vi "TARGET.vi"() -> ()   [LabVIEW 2018]
uses:
  <vilib>/Platform/TimedLoop/XDataNode/timing_clust.ctl
  <vilib>/Platform/TimedLoop/XDataNode/nitl_modes.ctl
  <vilib>/Platform/TimedLoop/XDataNode/wakeup.ctl
  <vilib>/rvi/eio/common/nirviEmuTemplateMethod_errors.vi
  <vilib>/rvi/Emulation/niFpgaGetClockAttributes.vi
  <vilib>/rvi/Emulation/niFpgaSctlEmulationGetInTimedLoop.vi
  <vilib>/rvi/Emulation/niFpgaEmulationReportErrorSimple.vi
  <vilib>/rvi/Emulation/niFpgaCriticalErrorInLSC.vi
  <vilib>/rvi/interface/RandomDataEmulation/niFpgaRandomDataHandleErrors.vi
  <vilib>/rvi/Emulation/niFpgaProcessEmulError.vi
  <vilib>/eio/EIONode/EIONode.xnode
  <vilib>/Platform/TimedLoop/XDataNode/XDataNode.xnode
  <vilib>/rvi/DataTransferAndStorage/Container/XNode/niFpgaContainer.xnode
  <vilib>/rvi/interface/RandomDataEmulation/nirviRandomDataFpgaReadWriteTemplate.vi
  <vilib>/Platform/TimedLoop/XDataNode/XDNodeRunTimeDep.lvlib
panel:
  in  "IO Module\\Local_Supply_Select":u8
  in  "IO Module\\DDCA_Supply_Select":bool=TRUE
  in  "8191?":u16=8191
  in  "Задержка, мкс":u16 caption="Count(mSec)"
  in  "50?":u16=50
  in  "Запись в FIFO":bool
  in  "HIGH":u8=18
  in  "LOW":u8=8
  in  "CLK_1":u16=59
  in  "ROG_1":u16=20
  in  "ROG_2":u16=40
  in  "SHUT1":u16=95
  in  "SHUT_2":u16=125
  in  "CLK_2":u8=9
  in  "CLK_3":u8=20
  in  "20":u8=20
  in  "42000?":u16=42000
  in  "П_41789?":u16=41789
  in  "ADC_2":u8=13
  in  "ADC_1":u8=2
  in  "CDS2_2":u8=15
  in  "CDS2_1":u8=10
  in  "CDS1_2":u8=9
  in  "CDS1_1":u8=2
  out "Данные":u8
  in  "Направление бит":bool
  in  "Линейки":bool
  in  "Остановка основного цикла":bool
  in  "Command array":bool[](array[boolean])=[FALSE, FALSE, FALSE, FALSE, FALSE, FALSE, FALSE, FALSE, FALSE, FALSE, FALSE, FALSE, FALSE, FALSE, FALSE, FALSE, FALSE]
  in  "Read(T)/Write(F)":bool
  in  "Enum":T1(ring)=enum."GREEN PGA"
  in  "Write Data":bool[](array[boolean])=[FALSE, FALSE, FALSE, FALSE, FALSE, FALSE, FALSE, FALSE, FALSE]
  out "READ":bool[](array[boolean])
  in  "Конфигурация":bool
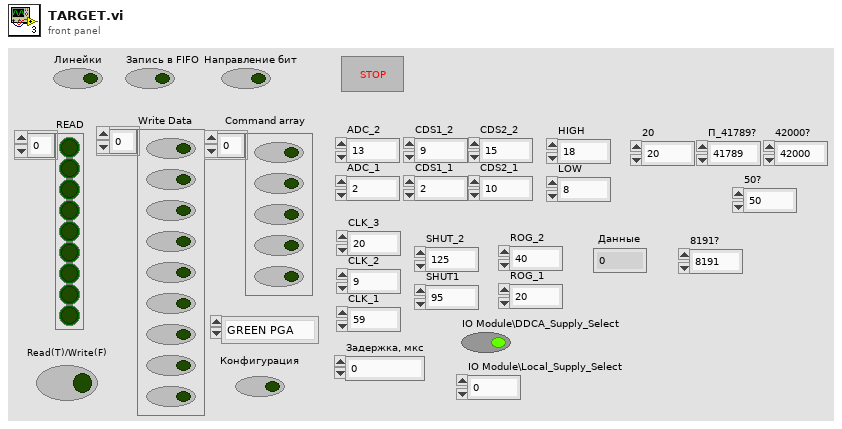
[diagram p1: front panel]
types:
  T1 = enum16{"Configuration", "MUX", "RED PGA", "GREEN PGA", "BLUE PGA", "RED OFF", "GREEN OFF", "BLUE OFF"}
  T2 = typedef "XDNodeRunTimeDep.lvlib/timing_clust.ctl" = cluster{"Expected End [f-1]":u64, "Actual End [f-1]":u64, "Finished Late? [f-1]":bool, "Expected End [i-1]":u64, "Actual End [i-1]":u64, "Finished Late? [i-1]":bool, "Expected Start [i]":u64, "Actual Start [i]":u64, "Expected Start [f]":u64, "Actual Start [f]":u64, "Source Name":string, "Structure Name":string, "Period":i64, "Deadline":i64, "Offset":i64, "Start":i64, "Priority":i32, "Timeout":i32, "Mode":T3, "Wakeup Reason":T4, "Error":errorcluster, "Source Type":string, "Secondary Source Type":string, "Global End Time":u64, "Global Start Time":u64, "Frame Duration":u64, "Iteration Duration":u64, "Assigned CPU":i32, "I/O Scan Engine Mode":u32}
  T3 = typedef "XDNodeRunTimeDep.lvlib/nitl_modes.ctl" = enum32{"No Change", "Process missed periods, maintain original phase", "Discard missed periods, maintain original phase", "Process missed periods, ignore original phase", "Discard missed periods, ignore original phase"}
  T4 = typedef "XDNodeRunTimeDep.lvlib/wakeup.ctl" = enum32{"Normal", "Aborted", "Asynchronous wakeup", "Timing source error", "Timed loop error", "Timeout"}
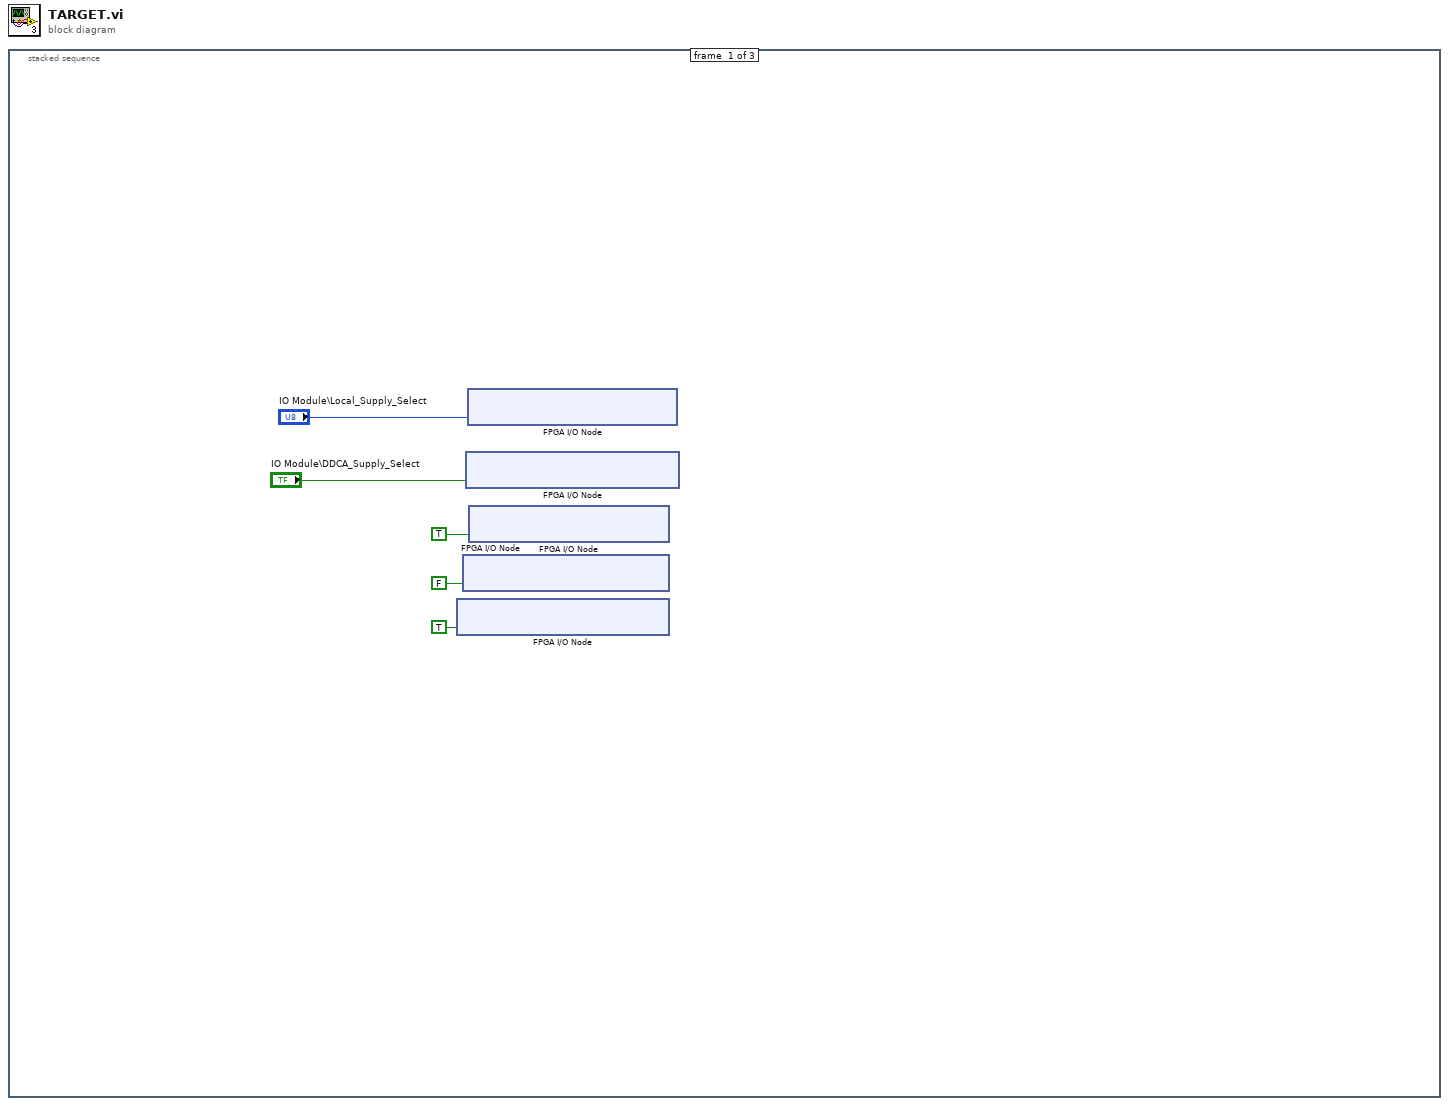
[diagram p0: block diagram]
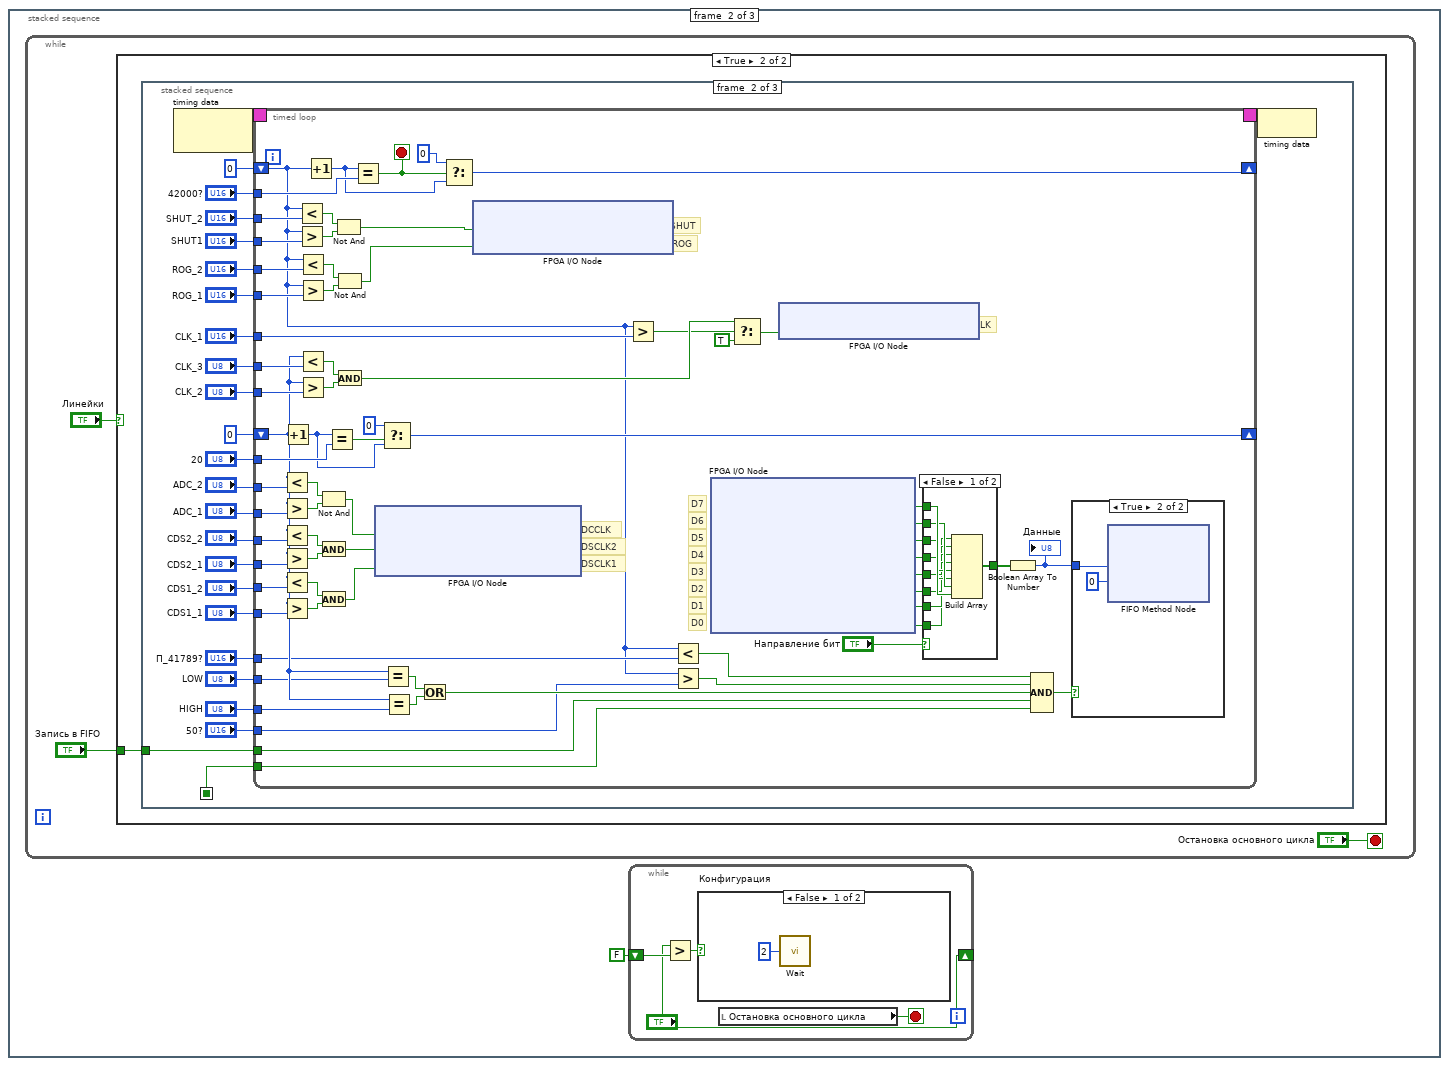
[diagram p2: hidden frame]
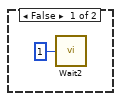
[diagram p3: hidden frame]
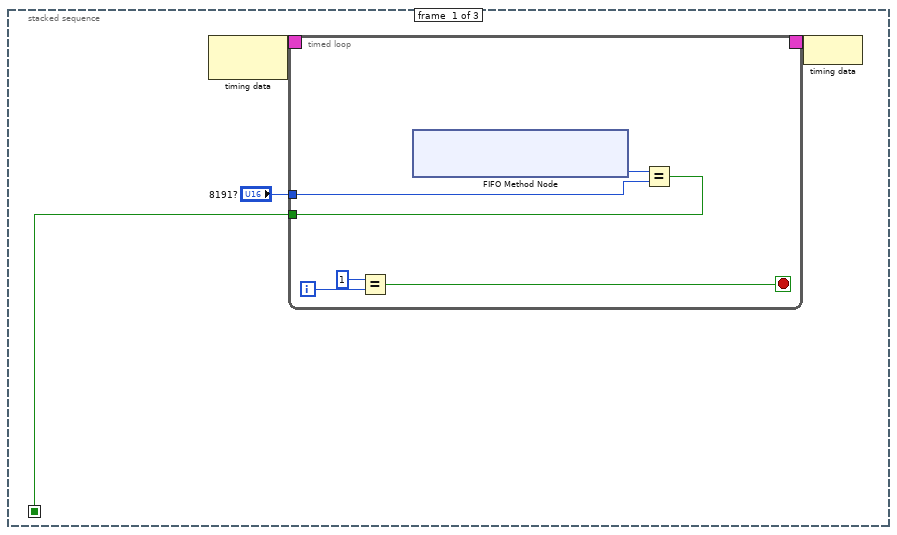
[diagram p4: hidden frame]
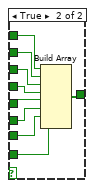
[diagram p6: hidden frame]
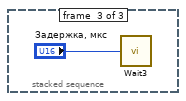
[diagram p7: hidden frame]
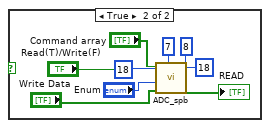
[diagram p8: hidden frame]
diagram:
  n1 = stacked-sequence {
    frame #0 {
      n2 = xnode "FPGA I/O Node"("IO Module\\DDCA_DIO16-23_WE"=TRUE) -> ()  [unwired: 1 in, 1 out]
      n3 = xnode "FPGA I/O Node"("IO Module\\DDCA_DIO8-15_WE"=FALSE) -> ()  [unwired: 1 in, 1 out]
      n4 = xnode "FPGA I/O Node"("IO Module\\DDCA_Supply_Select"="IO Module\\DDCA_Supply_Select") -> ()  [unwired: 1 in, 1 out]
      n5 = xnode "FPGA I/O Node"("IO Module\\Local_Supply_Select"="IO Module\\Local_Supply_Select") -> ()  [unwired: 1 in, 1 out]
      n6 = xnode "FPGA I/O Node"("IO Module\\DDCA_DIO0-7_WE"=TRUE) -> ()  [unwired: 1 in, 1 out]
    }
    frame #1 {
      n7 = while {
        stop <- "Остановка основного цикла" stop-if-true
        n8 = case shown="True" "Линейки" {
          tunnel: "Запись в FIFO" -> [_ w11]
          frame False {
            n9 = call "Wait2"("Count(Ticks)"=u8 1) -> ()  [unwired: 1 out]
          }
          frame True {
            n10 = stacked-sequence {
              seq-local: [w15 _ _] -> [_ w26 _]
              tunnel: w11 -> [_ w27 _]
              frame #0 {
                n11 = node-c288() -> (w14:T2)  [unwired: 1 in]
                n12 = timed-loop {
                  timing: w14 -> [_]
                  timing-out: [_] -> w13
                  tunnel: [w20] -> w15
                  tunnel: "8191?" -> [w16]
                  i -> [w19]
                  stop <- w17 stop-if-true
                  n13 = Equal?(x=1, y=w19) -> (x = y?=w17:bool)
                  n14 = xnode ("FIFO Method Node")() -> ("Number of Elements to Write"=w21:u32)  [unwired: 1 in, 1 out]
                  n15 = Equal?(x=w21, y=w16) -> (x = y?=w20:bool)
                }
                n16 = node-c288(w13) -> ()
              }
              frame #1 {
                n17 = node-c288() -> (w50:T2)  [unwired: 1 in]
                n18 = timed-loop {
                  timing: w50 -> [_]
                  timing-out: [_] -> w49
                  shift-right: [w71] -> _
                  shift-left: u16 0 -> [w55]
                  tunnel: "ADC_2" -> [w102]
                  tunnel: "ADC_1" -> [w101]
                  tunnel: "CDS2_2" -> [w100]
                  tunnel: "CDS2_1" -> [w99]
                  tunnel: "CDS1_2" -> [w98]
                  tunnel: "CDS1_1" -> [w97]
                  tunnel: "П_41789?" -> [w59]
                  tunnel: "42000?" -> [w75]
                  tunnel: "20" -> [w93]
                  shift-right: [w89] -> _
                  shift-left: u8 0 -> [w65]
                  tunnel: "CLK_3" -> [w82]
                  tunnel: "CLK_2" -> [w81]
                  tunnel: "SHUT_2" -> [w80]
                  tunnel: "SHUT1" -> [w79]
                  tunnel: "ROG_2" -> [w78]
                  tunnel: "ROG_1" -> [w77]
                  tunnel: "CLK_1" -> [w69]
                  tunnel: "LOW" -> [w64]
                  tunnel: "HIGH" -> [w63]
                  tunnel: "50?" -> [w54]
                  tunnel: w27 -> [w53]
                  tunnel: w26 -> [w51]
                  stop <- w72 stop-if-true
                  # "SHUT"
                  # "ROG"
                  # "CLK"
                  # "CDSCLK1"
                  # "CDSCLK2"
                  # "ADCCLK"
                  # "D0"
                  # "D1"
                  # "D2"
                  # "D3"
                  # "D4"
                  # "D5"
                  # "D6"
                  # "D7"
                  n19 = Less?(x=w65, y=w102) -> (x < y?=w103:bool)
                  n20 = Greater?(x=w65, y=w101) -> (0:w104:bool)
                  n21 = Less?(x=w65, y=w100) -> (x < y?=w106:bool)
                  n22 = Greater?(x=w65, y=w99) -> (0:w105:bool)
                  n23 = Less?(x=w65, y=w98) -> (x < y?=w107:bool)
                  n24 = Greater?(x=w65, y=w97) -> (0:w108:bool)
                  n25 = Increment(x=w65) -> (x+1=w90:u8)
                  n26 = Less?(x=w55, y=w80) -> (x < y?=w85:bool)
                  n27 = Greater?(x=w55, y=w79) -> (0:w86:bool)
                  n28 = Less?(x=w55, y=w78) -> (x < y?=w84:bool)
                  n29 = Greater?(x=w55, y=w77) -> (0:w83:bool)
                  n30 = Less?(x=w65, y=w82) -> (x < y?=w88:bool)
                  n31 = Greater?(x=w65, y=w81) -> (0:w87:bool)
                  n32 = Increment(x=w55) -> (x+1=w73:u16)
                  n33 = Not And(1:w104, 2:w103) -> (0:w96:bool)
                  n34 = And(x=w106, y=w105) -> (x .and. y?=w95:bool)
                  n35 = And(x=w107, y=w108) -> (x .and. y?=w94:bool)
                  n36 = Equal?(x=w90, y=w93) -> (x = y?=w92:bool)
                  n37 = Not And(1:w86, 2:w85) -> (0:w76:bool)
                  n38 = Not And(1:w83, 2:w84) -> (0:w70:bool)
                  n39 = And(x=w88, y=w87) -> (x .and. y?=w68:bool)
                  n40 = Equal?(x=w73, y=w75) -> (x = y?=w72:bool)
                  n41 = xnode "FPGA I/O Node"("IO Module\\DDCA_DIO16_Write"=w96, "IO Module\\DDCA_DIO17_Write"=w95, "IO Module\\DDCA_DIO18_Write"=w94) -> ()  [unwired: 3 in, 3 out]
                  n42 = Select(t=u8 0, s=w92, f=w90) -> (s? t:f=w89:u8)
                  n43 = Equal?(x=w65, y=w64) -> (x = y?=w61:bool)
                  n44 = Equal?(x=w65, y=w63) -> (x = y?=w62:bool)
                  n45 = Or(x=w61, y=w62) -> (x .or. y?=w60:bool)
                  n46 = Select(t=u16 0, s=w72, f=w73) -> (s? t:f=w71:u16)
                  n47 = xnode "FPGA I/O Node"("IO Module\\DDCA_DIO1_Write"=w76, "IO Module\\DDCA_DIO2_Write"=w70) -> ()  [unwired: 2 in, 2 out]
                  n48 = Greater?(x=w55, y=w69) -> (0:w58:bool)
                  n49 = Less?(x=w55, y=w59) -> (x < y?=w57:bool)
                  n50 = Greater?(x=w55, y=w54) -> (0:w56:bool)
                  n51 = xnode "FPGA I/O Node"() -> ("IO Module\\DDCA_DIO8_Read"=w116:bool, "IO Module\\DDCA_DIO9_Read"=w115:bool, "IO Module\\DDCA_DIO10_Read"=w114:bool, "IO Module\\DDCA_DIO11_Read"=w113:bool, "IO Module\\DDCA_DIO12_Read"=w112:bool, "IO Module\\DDCA_DIO13_Read"=w111:bool, "IO Module\\DDCA_DIO14_Read"=w110:bool, "IO Module\\DDCA_DIO15_Read"=w109:bool)  [unwired: 8 in, 8 out]
                  n52 = Select(t=w68, s=w58, f=TRUE) -> (s? t:f=w67:bool)
                  n53 = xnode "FPGA I/O Node"("IO Module\\DDCA_DIO0_Write"=w67) -> ()  [unwired: 1 in, 1 out]
                  n54 = case shown="False" "Направление бит" {
                    tunnel: w116 -> [w129 w139]
                    tunnel: w115 -> [w128 w138]
                    tunnel: w114 -> [w127 w137]
                    tunnel: w113 -> [w126 w136]
                    tunnel: w112 -> [w125 w135]
                    tunnel: w111 -> [w124 w134]
                    tunnel: w110 -> [w123 w133]
                    tunnel: w109 -> [w122 w132]
                    tunnel: [w130 w131] -> w119
                    frame False {
                      n55 = Build Array(w122, w123, w124, w125, w126, w127, w128, w129) -> (w130:bool[])
                    }
                    frame True {
                      n56 = Build Array(w139, w138, w137, w136, w135, w134, w133, w132) -> (w131:bool[])
                    }
                  }
                  n57 = Boolean Array To Number(Boolean array=w119) -> (number=w117:u8)
                  "Данные" <- w117
                  n58 = Compound Arithmetic op=AND(w57, w56, w60, w53, w51) -> (w52:bool)
                  n59 = case shown="True" w52 {
                    tunnel: w117 -> [_ w121]
                    frame False {
                    }
                    frame True {
                      n60 = xnode ("FIFO Method Node")("Element"=w121, "Timeout"=0) -> ()  [unwired: 1 in, 2 out]
                    }
                  }
                }
                n61 = node-c288(w49) -> ()
              }
              frame #2 {
                n62 = call "Wait3"("Count(uSec)"="Задержка, мкс") -> ()  [unwired: 1 out]
              }
            }
          }
        }
      }
      n63 = while {
        shift-right: ["Конфигурация"] -> _
        shift-left: FALSE ("Конфигурация") -> [w147]
        stop <- w148 stop-if-true
        n64 = Greater?(x="Конфигурация", y=w147) -> (0:w145:bool)
        n65 = case shown="False" w145 {
          frame False {
            n66 = call "Wait"("Count(Ticks)"=u8 2) -> ()  [unwired: 1 out]
          }
          frame True {
            n67 = call "ADC_spb.vi"(1:"18_1"=i8 18 ("18_1"), 2:"18_1"=i8 18 ("18_1"), "8"=i8 8, "7"=i8 7, "Write Data"="Write Data", "Enum"="Enum", "Read(T)/Write(F)"="Read(T)/Write(F)", "Command array"="Command array") -> ("READ"=→"READ":bool[])
          }
        }
        n68 = local read "Остановка основного цикла"() -> (w148:bool)
      }
    }
    frame #2 {
    }
  }
